vi "Read 32-Bit Word.vi"(8 "error in (no error)":errorcluster, 11 "32-bit Word in":refnum<class "32-bit Word.lvclass">) -> (0 "error out":errorcluster, 2 "32-bit word":u32 format="%032b", 3 "32-bit Word out":refnum<class "32-bit Word.lvclass">)   [LabVIEW 2020, in "32-bit Word.lvclass"]
uses:
  32-bit Word.lvclass
  32-bit Word.lvclass/32-bit Word.ctl
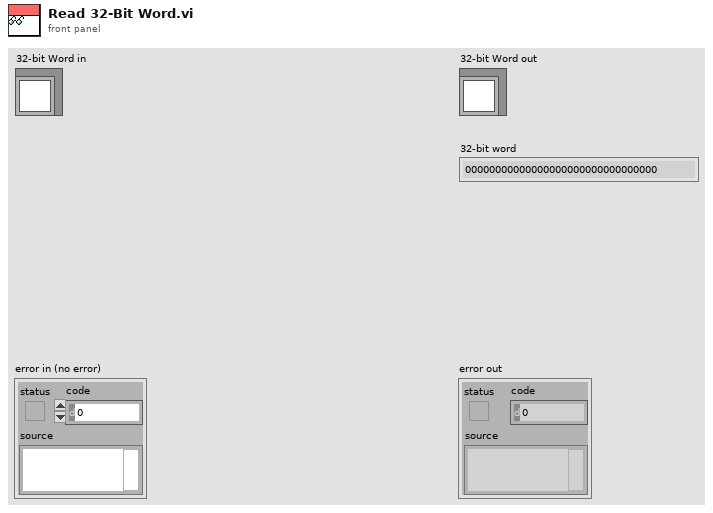
[diagram p1: front panel]
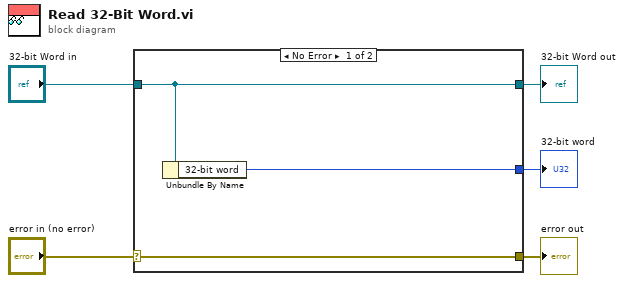
[diagram p0: block diagram]
diagram:
  n1 = case shown="No Error" "error in (no error)" {
    selector: "error in (no error)" -> [w8 w9]
    tunnel: [w8 w9] -> w4
    tunnel: [w7 w10] -> w2
    tunnel: "32-bit Word in" -> [w7 w10]
    tunnel: [w6 _] -> w1
    frame No Error {
      n2 = Unbundle By Name(w7) -> ("32-bit word"=w6:u32)
    }
    frame Error {
    }
  }
  "error out" <- w4
  "32-bit Word out" <- w2
  "32-bit word" <- w1
